vi "Write Wash Entry Ref.vi"(6 "Wash Entry Ref":refnum<vi>, 11 "Car Wash Status View Definition in":refnum<class "Car Wash Status View Definition.lvclass">) -> (3 "Car Wash Status View Definition out":refnum<class "Car Wash Status View Definition.lvclass">)   [LabVIEW 2019, in "Car Wash Status View Definition.lvclass"]
uses:
  <vilib>/gpm_packages/@cs/Car-wash/Source/Car Wash Status View Definition/Car Wash Status View Definition/Car Wash Status View Definition.lvclass
  <vilib>/gpm_packages/@cs/Car-wash/Source/Car Wash Status View Definition/Car Wash Status View Definition/Car Wash Status View Definition.lvclass/Car Wash Status View Definition.ctl
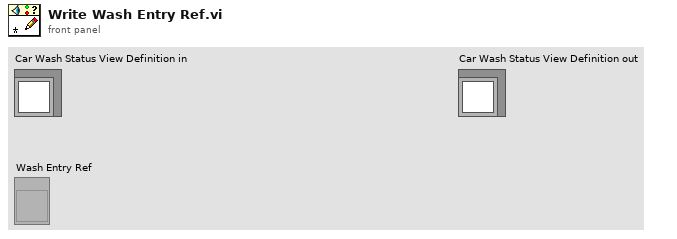
[diagram p1: front panel]
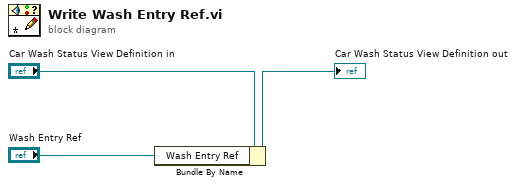
[diagram p0: block diagram]
diagram:
  n1 = Bundle By Name(cluster="Car Wash Status View Definition in", "Wash Entry Ref"="Wash Entry Ref") -> (→"Car Wash Status View Definition out":refnum<class "Car Wash Status View Definition.lvclass">)
